vi "NF WF1973_74 OFFS User.vi"(0 "VISAsession":refnum<visa-resource-name>, 1 "Type(LIN)":u16(ring) items=["Linear", "Logarithmic"], 5 "Ch(Ch1)":bool, 9 "Unit Name(DEFA)":string="DEFA", 11 "error in (no error)":errorcluster caption="Error IN", 12 "Read(F)":bool, 13 "Scale(0)":dbl format="%.2f", 14 "Offset(0)":dbl format="%.2f") -> (4 "CopyVISAsession":refnum<visa-resource-name>, 6 "Query Unit":string, 15 "error out":errorcluster caption="Error OUT")   [LabVIEW 2010]
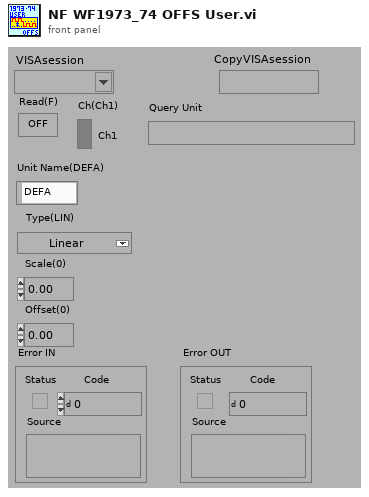
[diagram p1: front panel]
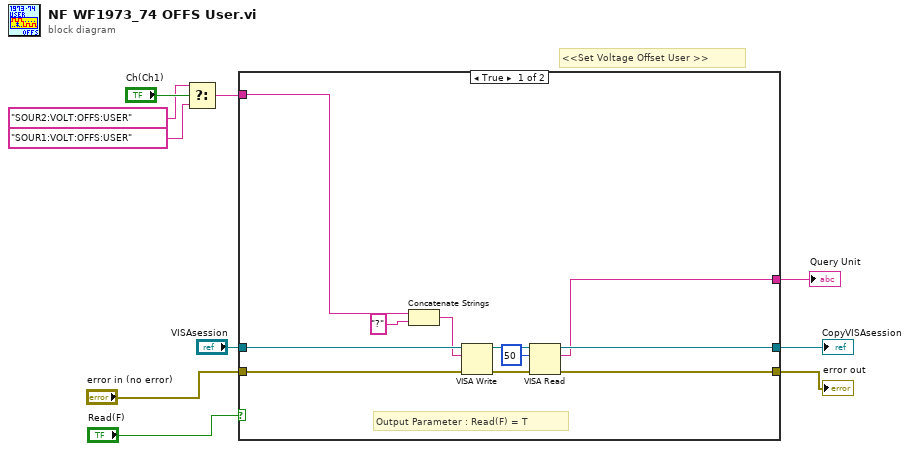
[diagram p0: block diagram]
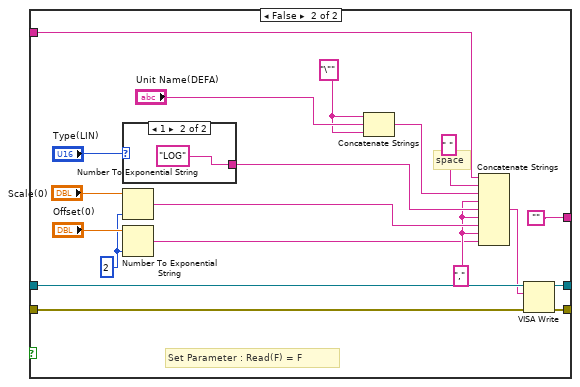
[diagram p2: hidden frame]
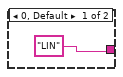
[diagram p3: hidden frame]
diagram:
  # "<<Set Voltage Offset User >>"
  n1 = Select(t="SOUR2:VOLT:OFFS:USER" ("文字列"), s="Ch(Ch1)", f="SOUR1:VOLT:OFFS:USER" ("文字列")) -> (s? t:f=w4:string)
  n2 = case shown="TRUE" "Read(F)" {
    tunnel: "VISAsession" -> [w21 w40]
    tunnel: [w18 w38] -> w9
    tunnel: [w17 w39] -> w8
    tunnel: "error in (no error)" -> [w16 w35]
    tunnel: w4 -> [w14 w36]
    tunnel: [w11 ""] -> w1
    frame True {
      # "Output Parameter : Read(F) = T"
      n3 = Concatenate Strings(w14, "?" ("形式文字列")) -> (w12:string)
      n4 = VISA Write(VISA resource name=w21, write buffer=w12, error in (no error)=w16) -> (VISA resource name out=w19:refnum<visa-resource-name>, error out=w20:errorcluster)  [unwired: 1 out]
      n5 = VISA Read(VISA resource name=w19, byte count=u32 50 ("バイトカウント（0）"), error in (no error)=w20) -> (VISA resource name out=w18:refnum<visa-resource-name>, read buffer=w11:string, error out=w17:errorcluster)  [unwired: 1 out]
    }
    frame False {
      w25 = i16 2 ("精度 (6)")
      w22 = "\""
      w27 = ","
      # "space"
      # "Set Parameter : Read(F) = F"
      n6 = case shown="1" "Type(LIN)" {
        tunnel: ["LIN" "LOG"] -> w29
        frame 0, Default {
        }
        frame 1 {
        }
      }
      n7 = Number To Exponential String(number="Scale(0)", precision (6)=w25) -> (E-format string=w28:string)  [unwired: 2 in]
      n8 = Number To Exponential String(number="Offset(0)", precision (6)=w25) -> (E-format string=w26:string)  [unwired: 2 in]
      n9 = Concatenate Strings(w22, "Unit Name(DEFA)", w22) -> (w23:string)
      n10 = Concatenate Strings(w36, " ", w23, w27, w29, w27, w28, w27, w26) -> (w37:string)
      n11 = VISA Write(VISA resource name=w40, write buffer=w37, error in (no error)=w35) -> (VISA resource name out=w38:refnum<visa-resource-name>, error out=w39:errorcluster)  [unwired: 1 out]
    }
  }
  "error out" <- w8
  "CopyVISAsession" <- w9
  "Query Unit" <- w1
